vi "RT-sigmoid.vi"(1 "x":dbl) -> (0 "Sigmoid":dbl)   [LabVIEW 2020]
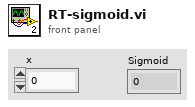
[diagram p1: front panel]
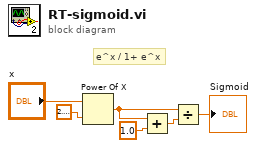
[diagram p0: block diagram]
diagram:
  # "e^x / 1+ e^x"
  n1 = Power Of X(1:2.718281828459045, 2:"x") -> (0:w3:dbl)
  n2 = Add(x=w3, y=1.0) -> (x+y=w2:dbl)
  n3 = Divide(x=w3, y=w2) -> (x/y=→"Sigmoid":dbl)
